vi "Periodic Tasks.vi"(8 "error in":errorcluster) -> ()   [LabVIEW 2012]
doc: "This VI runs in parallel to other tasks. It can contain as many user-defined periodic loops as you need. These can carry out PID or other sorts of timed response."
uses:
  <vilib>/Rock Robotics/SystemInterfaces/Utilities/FPGA_UtilitiesLED Source.ctl
  <vilib>/Rock Robotics/SystemInterfaces/Utilities/FPGA_UtilitiesLED State.ctl
  <vilib>/Rock Robotics/WPI/RobotDrive/WPI_RobotDriveGetSetRefNum.vi
  Robot Global Data.vi
  <vilib>/Rock Robotics/WPI/Joystick/WPI_JoystickGetSetRefNum.vi
  <vilib>/addons/control/pid/pid.llb/PID (DBL).vi
  <vilib>/addons/control/pid/NI_PID_pid.lvlib
panel:
  in  "setpoint 4":dbl=1500.0 format="%.2f"
  in  "setpoint 3":dbl=1500.0 format="%.2f"
  in  "PID gains 3":T1={"proportional gain (Kc)"=0.01, "integral time (Ti, min)"=0.0, "derivative time (Td, min)"=0.0}
  in  "PID gains 2":T1={"proportional gain (Kc)"=0.01, "integral time (Ti, min)"=0.0, "derivative time (Td, min)"=0.0}
  in  "PID gains":T1={"proportional gain (Kc)"=0.01, "integral time (Ti, min)"=0.0, "derivative time (Td, min)"=0.0}
  in  "setpoint":dbl=1500.0 format="%.2f"
  in  "setpoint 2":dbl=1500.0 format="%.2f"
  in  "Accel Rate":dbl=0.1
  in  "error in 2":errorcluster
  out "Sonar Distance Average":dbl
  out "Sonar Distance Output":dbl
  out "Sonar Voltage":dbl
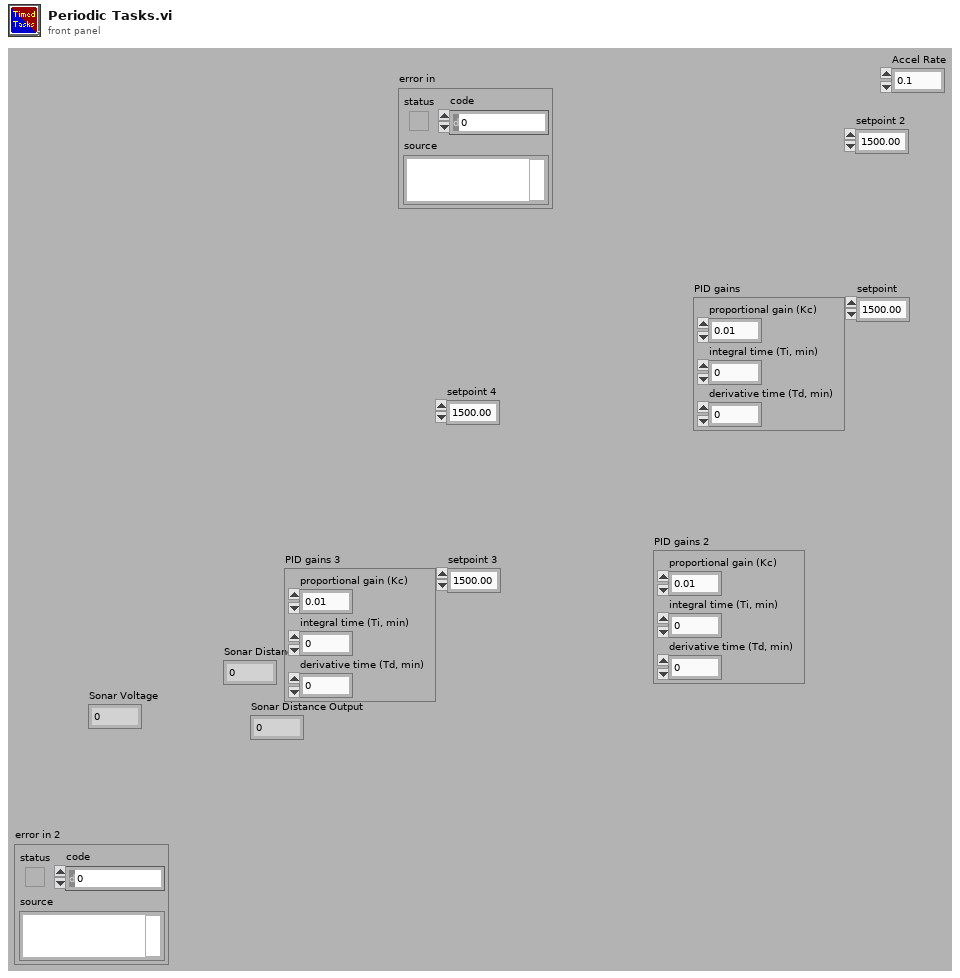
[diagram p1: front panel]
types:
  T1 = cluster{"proportional gain (Kc)":dbl, "integral time (Ti, min)":dbl, "derivative time (Td, min)":dbl}
  T2 = typedef "WPI_JoystickDevRef.ctl" = cluster{"Device":T3}
  T3 = typedef "WPI_JoystickDeviceEnum.ctl" = enum16{"USB 1", "USB 2", "USB 3", "USB 4", "Kinect 1", "Kinect 2"}
  T4 = typedef "WPI_RobotDriveDevRef.ctl" = cluster{"DevStatus":errorcluster, "Motors[]":T5[], "Square Inputs":bool, "Max Output":dbl, "Isochronous":bool}
  T5 = typedef "WPI_MotorControlDeviceRef.ctl" = cluster{"DeviceStatus":errorcluster, "Type":enum16{"PWM", "CAN"}, "PWM":cluster{"Digital Module":T6, "PWM Channel":T7, "DeadBand":T8}, "CAN":cluster{"Device Number":u8, "Control Mode":T9, "Semaphore":T10, "Max Vout":dbl}, "Invert":bool, "TransformRef":T11, "InvTransformRef":T11}
  T6 = typedef "FPGA_TypedefDigitalModule.ctl" = enum16{"Digital Module 1", "Digital Module 2"}
  T7 = typedef "FPGA_DIOPWMChannel.ctl" = enum8{"PWM 1", "PWM 2", "PWM 3", "PWM 4", "PWM 5", "PWM 6", "PWM 7", "PWM 8", "PWM 9", "PWM 10", "Invalid"}
  T8 = typedef "WPI_PWMDeadband.ctl" = cluster{"Name":string, "maxPositivePwm":i32, "minPositivePwm":i32, "centerPwm":i32, "maxNegativePwm":i32, "minNegativePwm":i32, "angularRange":u16}
  T9 = typedef "WPI_CANJaguar_ControlMode.ctl" = enum8{"Percent VBus", "Current", "Speed", "Position", "Voltage"}
  T10 = typedef "Semaphore RefNum" = refnum<k1>
  T11 = typedef "WPI_PWMTransform_ConPane.ctl" = refnum<vi>
  T12 = cluster{"JoystickDevRef":T2, "RobotDriveDevRef":T4, "RobotDriveDevRef":T4}
  T13 = cluster{"axis 1 (x)":dbl, "axis 2 (y)":dbl, "axis 3 (throttle)":dbl, "axis 4":dbl, "axis 5":dbl, "axis 6":dbl}
  T14 = typedef "WPI_AnalogChannelDevRef.ctl" = cluster{"DevStatus":errorcluster, "Analog Module":T15, "Analog Channel":T16}
  T15 = typedef "FPGA_TypedefAnalogModule.ctl" = enum16{"Analog Module 1", "Analog Module 2"}
  T16 = typedef "FPGA_AIChannel.ctl" = enum8{"AI 1", "AI 2", "AI 3", "AI 4", "AI 5", "AI 6", "AI 7", "AI 8", "Invalid"}
  T17 = typedef "WPI_DigitalOutputDevRef.ctl" = cluster{"Digital Module":T6, "DIO Channel":T18, "DevStatus":errorcluster}
  T18 = typedef "FPGA_DIOChannel.ctl" = enum8{"DIO 1", "DIO 2", "DIO 3", "DIO 4", "DIO 5", "DIO 6", "DIO 7", "DIO 8", "DIO 9", "DIO 10", "DIO 11", "DIO 12", "DIO 13", "DIO 14", "Invalid"}
  T19 = typedef "WPI_JoystickButtonState.ctl" = cluster{"Button 1":bool, "Button 2":bool, "Button 3":bool, "Button 4":bool, "Button 5":bool, "Button 6":bool, "Button 7":bool, "Button 8":bool, "Button 9":bool, "Button 10":bool, "Button 11":bool, "Button 12":bool}
  T20 = typedef "FPGA_UtilitiesLED State.ctl" = enum16{"Off", "On", "Toggle"}
  T21 = typedef "FPGA_UtilitiesLED Source.ctl" = enum16{"User LED", "FPGA LED"}
  T22 = typedef "WPI_EncoderDevRef.ctl" = cluster{"DevStatus":errorcluster, "EncoderIndex":T23, "CounterIndex":T24, "DistancePerCount":dbl, "Decoding Type":T25}
  T23 = typedef "FPGA_EncoderIdx.ctl" = enum8{"Enc 0", "Enc 1", "Enc 2", "Enc 3", "Invalid"}
  T24 = typedef "FPGA_CounterCtrSystemIndex.ctl" = enum8{"Ctr 0", "Ctr 1", "Ctr 2", "Ctr 3", "Ctr 4", "Ctr 5", "Ctr 6", "Ctr 7", "Invalid"}
  T25 = typedef "WPI_EncoderType.ctl" = enum16{"1x", "2x", "4x"}
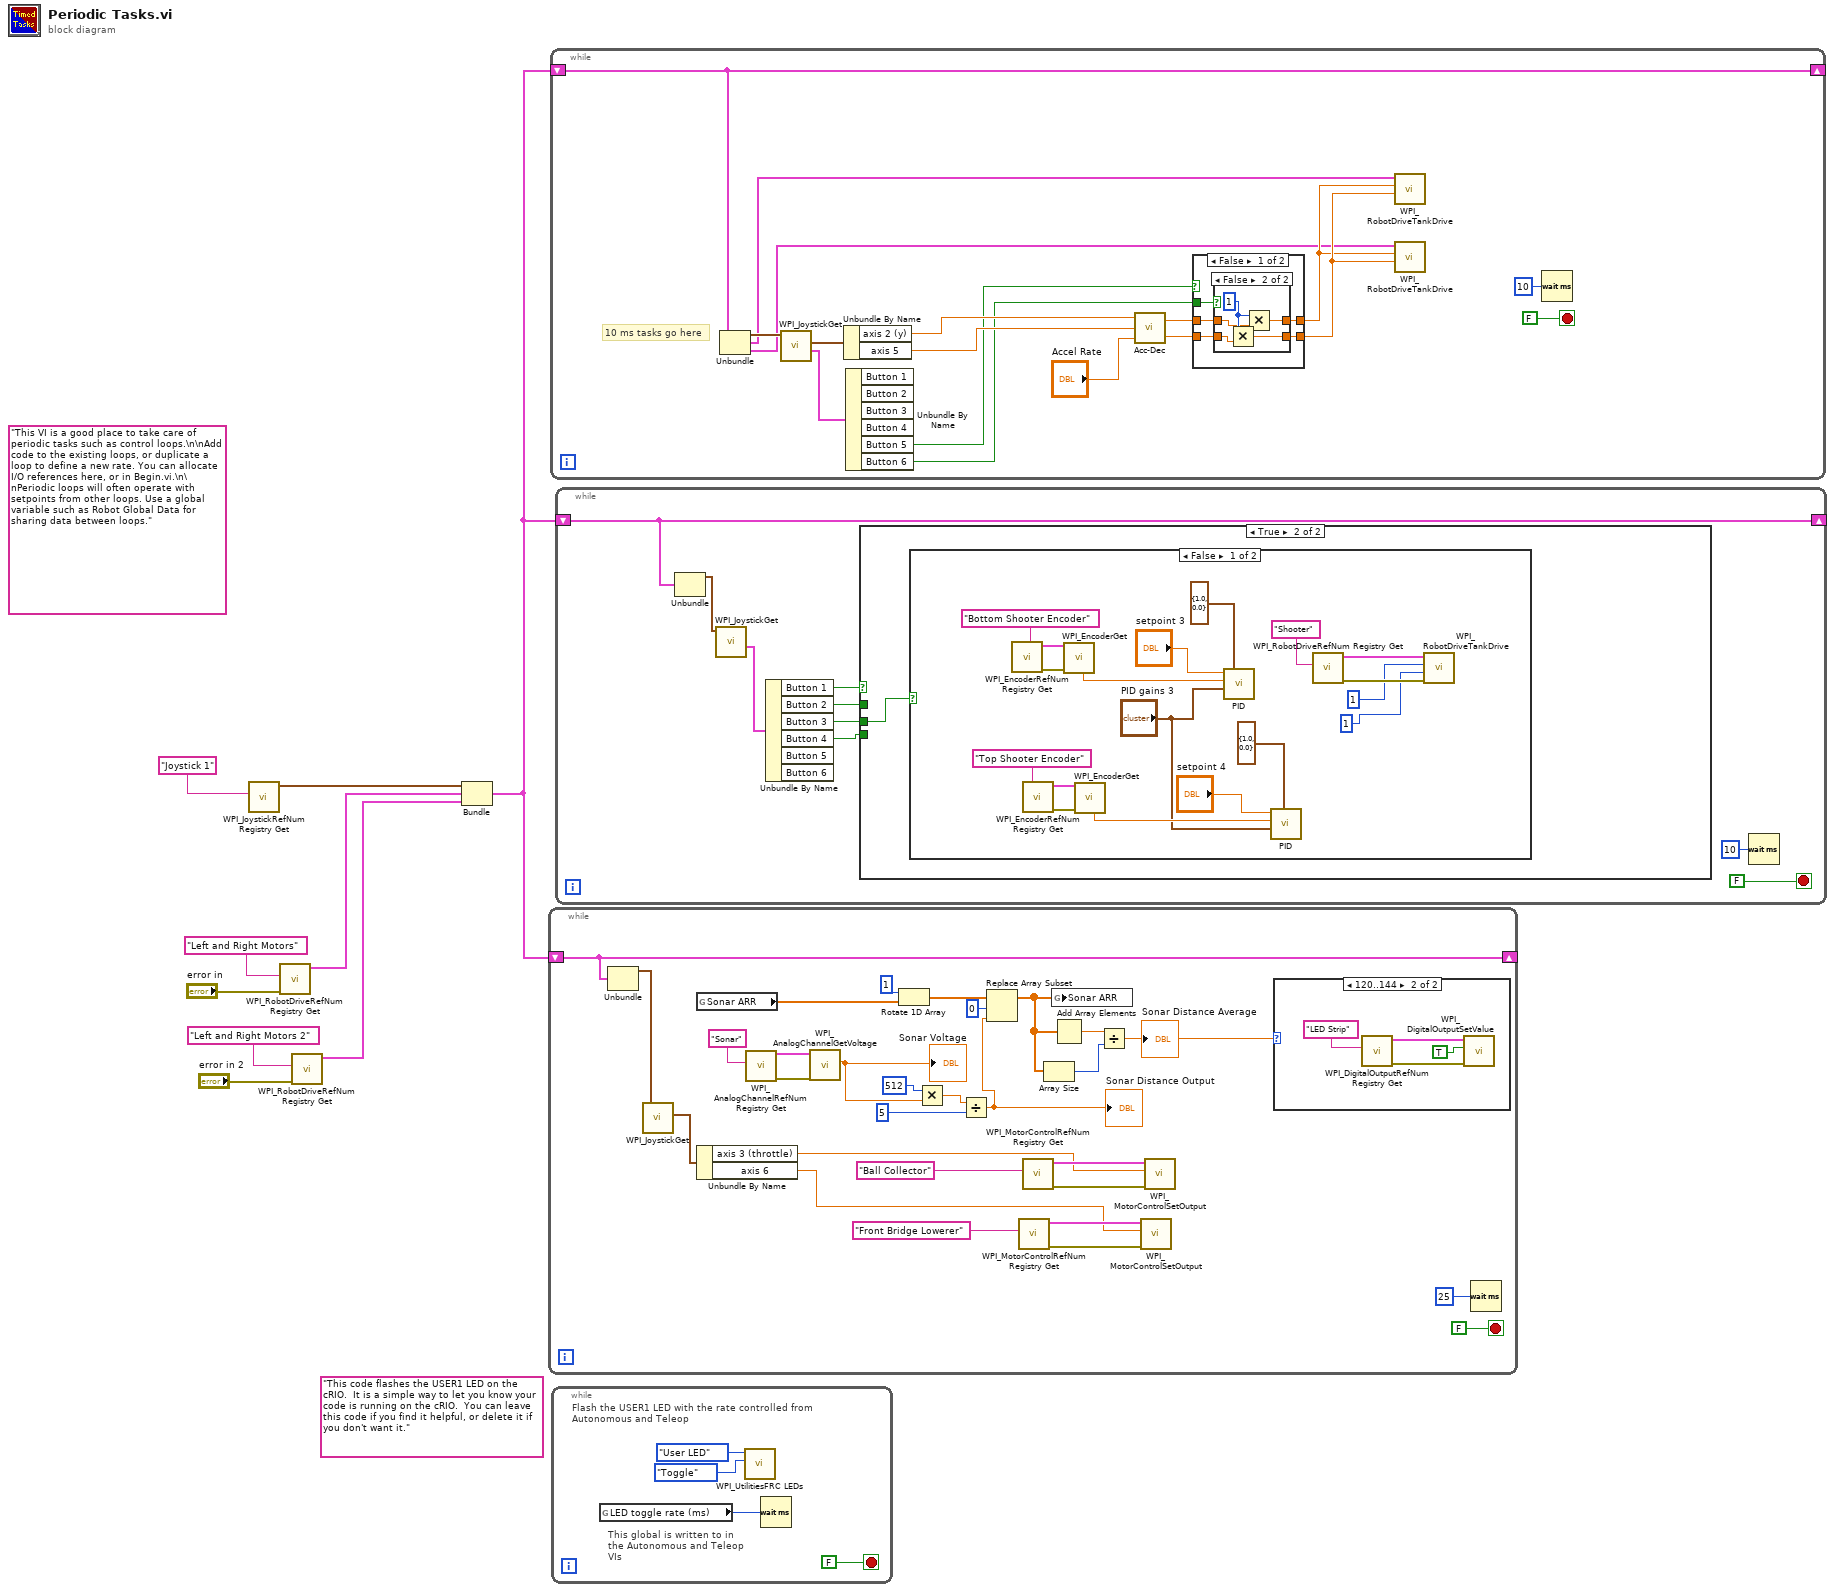
[diagram p0: block diagram]
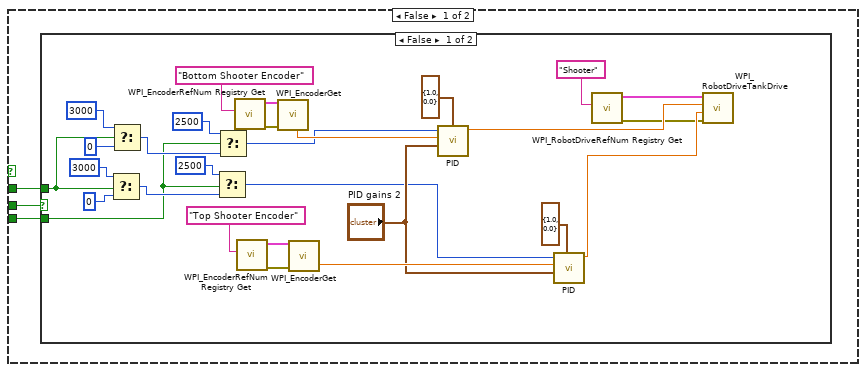
[diagram p2: hidden frame]
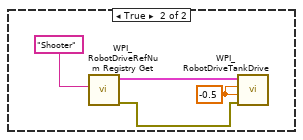
[diagram p3: hidden frame]
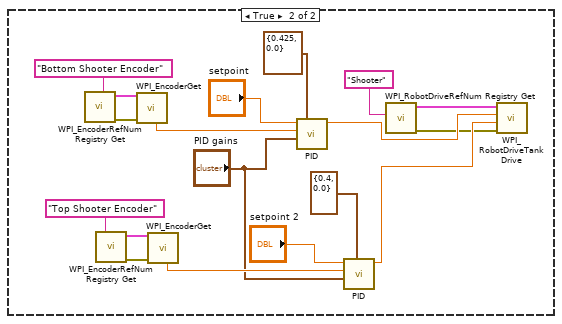
[diagram p4: hidden frame]
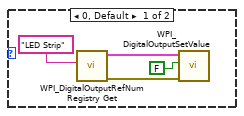
[diagram p5: hidden frame]
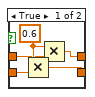
[diagram p6: hidden frame]
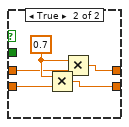
[diagram p7: hidden frame]
diagram:
  (unwired) "This code flashes the USER1 LED on the cRIO.  It is a simple way to let you know your code is running on the cRIO.  You can leave this code if you find it helpful, or delete it if you don't want it."
  (unwired) "This VI is a good place to take care of periodic tasks such as control loops.\n\nAdd code to the existing loops, or duplicate a loop to define a new rate. You can allocate I/O references here, or in Begin.vi.\n\nPeriodic loops will often operate with setpoints from other loops. Use a global variable such as Robot Global Data for sharing data between loops."
  n1 = call <vilib>:"WPI_JoystickRefNum Registry Get.vi"("refnum name"="Joystick 1") -> ("JoystickDevRef"=w7:T2)  [unwired: 1 in, 9 out]
  n2 = call <vilib>:"WPI_RobotDriveRefNum Registry Get.vi"("error in (no error)"="error in", "refnum name"="Left and Right Motors") -> ("RobotDriveDevRef"=w6:T4)  [unwired: 9 out]
  n3 = call <vilib>:"WPI_RobotDriveRefNum Registry Get.vi"("error in (no error)"="error in 2", "refnum name"="Left and Right Motors 2") -> ("RobotDriveDevRef"=w2:T4)  [unwired: 9 out]
  n4 = Bundle("JoystickDevRef"=w7, "RobotDriveDevRef"=w6, "RobotDriveDevRef"=w2) -> (w1:T12)  [unwired: 1 out]
  n5 = while {
    shift-right: [w20] -> _
    shift-left: w1 -> [w20]
    stop <- FALSE stop-if-true
    n6 = Unbundle(w20) -> ("JoystickDevRef"=w18:T2)  [unwired: 2 out]
    n7 = call <vilib>:"WPI_JoystickGet.vi"("JoystickDevRef"=w18) -> ("Axes"=w19:T13)  [unwired: 1 in, 5 out]
    n8 = global read "Robot Global Data.vi" "Sonar ARR"() -> (w31:dbl[])
    n9 = Unbundle By Name(w19) -> ("axis 3 (throttle)"=w10:dbl, "axis 6"=w14:dbl)
    n10 = call <vilib>:"WPI_AnalogChannelRefNum Registry Get.vi"("refnum name"="Sonar") -> ("error out"=w23:errorcluster, "AIDeviceRef"=w33:T14)  [unwired: 9 in]
    n11 = call <vilib>:"WPI_AnalogChannelGetVoltage.vi"("error in (no error)"=w23, "AIDeviceRef"=w33) -> ("Voltage"=w32:dbl)  [unwired: 7 in, 2 out]
    "Sonar Voltage" <- w32
    n12 = Rotate 1D Array(1:w31, 2:1) -> (0:w29:dbl[])
    n13 = Multiply(x=512, y=w32) -> (x*y=w35:dbl)
    n14 = Divide(x=w35, y=5) -> (x/y=w28:dbl)
    "Sonar Distance Output" <- w28
    n15 = Replace Array Subset(array=w29, new element=w28, index=0) -> (w25:dbl[])
    n16 = call <vilib>:"WPI_MotorControlRefNum Registry Get.vi"("refnum name"="Front Bridge Lowerer") -> ("error out"=w16:errorcluster, "MotorControlDevRef"=w15:T5)  [unwired: 9 in]
    n17 = call <vilib>:"WPI_MotorControlRefNum Registry Get.vi"("refnum name"="Ball Collector") -> ("error out"=w12:errorcluster, "MotorControlDevRef"=w11:T5)  [unwired: 9 in]
    n18 = Array Size(array=w25) -> (size(s)=w24:i32)
    n19 = global write "Robot Global Data.vi" "Sonar ARR"(w25) -> ()
    n20 = Add Array Elements(numeric array=w25) -> (sum=w26:dbl)
    n21 = Divide(x=w26, y=w24) -> (x/y=w22:dbl)
    "Sonar Distance Average" <- w22
    n22 = call <vilib>:"WPI_MotorControlSetOutput.vi"("error in (no error)"=w16, "Output"=w14, "MotorControlDevRef"=w15) -> ()  [unwired: 6 in, 3 out]
    n23 = call <vilib>:"WPI_MotorControlSetOutput.vi"("error in (no error)"=w12, "Output"=w10, "MotorControlDevRef"=w11) -> ()  [unwired: 6 in, 3 out]
    n24 = case shown="120..144" w22 {
      frame 0, Default {
        n25 = call <vilib>:"WPI_DigitalOutputRefNum Registry Get.vi"("refnum name"="LED Strip") -> ("error out"=w40:errorcluster, "DigitalOutputDevRef"=w41:T17)  [unwired: 9 in]
        n26 = call <vilib>:"WPI_DigitalOutputSetValue.vi"("error in (no error)"=w40, "Value"=FALSE, "DigitalOutputDevRef"=w41) -> ()  [unwired: 7 in, 2 out]
      }
      frame 120..144 {
        n27 = call <vilib>:"WPI_DigitalOutputRefNum Registry Get.vi"("refnum name"="LED Strip") -> ("error out"=w44:errorcluster, "DigitalOutputDevRef"=w45:T17)  [unwired: 9 in]
        n28 = call <vilib>:"WPI_DigitalOutputSetValue.vi"("error in (no error)"=w44, "Value"=TRUE, "DigitalOutputDevRef"=w45) -> ()  [unwired: 7 in, 2 out]
      }
    }
    n29 = Wait (ms)(milliseconds to wait=u32 25) -> ()  [unwired: 1 out]
  }
  n30 = while {
    shift-right: [w61] -> _
    shift-left: w1 -> [w61]
    stop <- FALSE stop-if-true
    # "10 ms tasks go here"
    n31 = Unbundle(w61) -> ("JoystickDevRef"=w58:T2, "RobotDriveDevRef"=w55:T4, "RobotDriveDevRef"=w54:T4)
    n32 = call <vilib>:"WPI_JoystickGet.vi"("JoystickDevRef"=w58) -> ("Buttons"=w59:T19, "Axes"=w60:T13)  [unwired: 1 in, 4 out]
    n33 = Unbundle By Name(w60) -> ("axis 2 (y)"=w51:dbl, "axis 5"=w52:dbl)
    n34 = Unbundle By Name(w59) -> ("Button 5"=w47:bool, "Button 6"=w48:bool)  [unwired: 4 out]
    n35 = call "Acc-Dec.vi"("Acc Rate"="Accel Rate", "Y-Input 2"=w52, "Y-Input 1"=w51) -> ("Y-Output 2"=w49:dbl, "Y-Output 1"=w50:dbl)
    n36 = case shown="False" w47 {
      tunnel: [w68 w79] -> w57
      tunnel: [w67 w80] -> w56
      tunnel: w50 -> [w66 w81]
      tunnel: w49 -> [w65 w82]
      tunnel: w48 -> [w64 _]
      frame False {
        n37 = case shown="False" w64 {
          tunnel: [w71 w76] -> w67
          tunnel: w66 -> [w69 w74]
          tunnel: [w73 w78] -> w68
          tunnel: w65 -> [w72 w77]
          frame True {
            w70 = 0.6
            n38 = Multiply(x=w70, y=w72) -> (x*y=w73:dbl)
            n39 = Multiply(x=w70, y=w69) -> (x*y=w71:dbl)
          }
          frame False {
            w75 = 1
            n40 = Multiply(x=w75, y=w77) -> (x*y=w78:dbl)
            n41 = Multiply(x=w75, y=w74) -> (x*y=w76:dbl)
          }
        }
      }
      frame True {
        w83 = 0.7
        n42 = Multiply(x=w83, y=w82) -> (x*y=w79:dbl)
        n43 = Multiply(x=w83, y=w81) -> (x*y=w80:dbl)
      }
    }
    n44 = call <vilib>:"WPI_RobotDriveTankDrive.vi"("Right axis value"=w57, "Left axis value"=w56, "RobotDriveDevRef"=w55) -> ()  [unwired: 6 in, 3 out]
    n45 = call <vilib>:"WPI_RobotDriveTankDrive.vi"("Right axis value"=w57, "Left axis value"=w56, "RobotDriveDevRef"=w54) -> ()  [unwired: 6 in, 3 out]
    n46 = Wait (ms)(milliseconds to wait=u32 10) -> ()  [unwired: 1 out]
  }
  n47 = while {
    stop <- FALSE stop-if-true
    # "This global is written to in the Autonomous and Teleop VIs"
    # "Flash the USER1 LED with the rate controlled from Autonomous and Teleop"
    n48 = global read "Robot Global Data.vi" "LED toggle rate (ms)"() -> (w84:u32)
    n49 = call <vilib>:"WPI_UtilitiesFRC LEDs.vi"("State"=FPGA_UtilitiesLED_State."Toggle", "LED Type"=FPGA_UtilitiesLED_Source."User LED") -> ()  [unwired: 1 in, 9 out]
    n50 = Wait (ms)(milliseconds to wait=w84) -> ()  [unwired: 1 out]
  }
  n51 = while {
    shift-right: [w96] -> _
    shift-left: w1 -> [w96]
    stop <- FALSE stop-if-true
    n52 = Unbundle(w96) -> ("JoystickDevRef"=w94:T2)  [unwired: 2 out]
    n53 = call <vilib>:"WPI_JoystickGet.vi"("JoystickDevRef"=w94) -> ("Buttons"=w95:T19)  [unwired: 1 in, 5 out]
    n54 = Unbundle By Name(w95) -> ("Button 1"=w93:bool, "Button 2"=w89:bool, "Button 3"=w92:bool, "Button 4"=w88:bool)  [unwired: 2 out]
    n55 = case shown="True" w93 {
      tunnel: w92 -> [w99 w132]
      tunnel: w89 -> [w98 _]
      tunnel: w88 -> [w97 _]
      frame False {
        n56 = case shown="False" w99 {
          tunnel: w98 -> [w108 _]
          tunnel: w97 -> [w103 _]
          frame False {
            n57 = Select(t=3000, s=w108, f=0) -> (s? t:f=w104:i32)
            n58 = Select(t=3000, s=w108, f=0) -> (s? t:f=w105:i32)
            n59 = Select(t=2500, s=w103, f=w104) -> (s? t:f=w102:i32)
            n60 = Select(t=2500, s=w103, f=w105) -> (s? t:f=w101:i32)
            n61 = call <vilib>:"WPI_EncoderRefNum Registry Get.vi"("refnum name"="Bottom Shooter Encoder") -> ("error out"=w120:errorcluster, "EncoderDevRef"=w121:T22)  [unwired: 9 in]
            n62 = call <vilib>:"WPI_EncoderRefNum Registry Get.vi"("refnum name"="Top Shooter Encoder") -> ("error out"=w123:errorcluster, "EncoderDevRef"=w124:T22)  [unwired: 9 in]
            n63 = call <vilib>:"WPI_EncoderGet.vi"("error in (no error)"=w120, "EncoderDevRef"=w121) -> ("Rate"=w118:dbl)  [unwired: 4 in, 5 out]
            n64 = call <vilib>:"WPI_EncoderGet.vi"("error in (no error)"=w123, "EncoderDevRef"=w124) -> ("Rate"=w117:dbl)  [unwired: 4 in, 5 out]
            n65 = call-poly <vilib>:"PID.vi"("output range"=cluster{"output high":dbl, "output low":dbl} {"output high"=1.0, "output low"=0.0}, "PID gains"="PID gains 2", "process variable"=w118, "setpoint"=w101) -> ("output"=w115:dbl)  [unwired: 6 in, 1 out]
            n66 = call-poly <vilib>:"PID.vi"("output range"=cluster{"output high":dbl, "output low":dbl} {"output high"=1.0, "output low"=0.0}, "PID gains"="PID gains 2", "process variable"=w117, "setpoint"=w102) -> ("output"=w116:dbl)  [unwired: 6 in, 1 out]
            n67 = call <vilib>:"WPI_RobotDriveRefNum Registry Get.vi"("refnum name"="Shooter") -> ("error out"=w100:errorcluster, "RobotDriveDevRef"=w127:T4)  [unwired: 1 in, 8 out]
            n68 = call <vilib>:"WPI_RobotDriveTankDrive.vi"("error in (no error)"=w100, "Right axis value"=w116, "Left axis value"=w115, "RobotDriveDevRef"=w127) -> ()  [unwired: 5 in, 3 out]
          }
          frame True {
            w129 = -0.5
            n69 = call <vilib>:"WPI_RobotDriveRefNum Registry Get.vi"("refnum name"="Shooter") -> ("error out"=w128:errorcluster, "RobotDriveDevRef"=w130:T4)  [unwired: 1 in, 8 out]
            n70 = call <vilib>:"WPI_RobotDriveTankDrive.vi"("error in (no error)"=w128, "Right axis value"=w129, "Left axis value"=w129, "RobotDriveDevRef"=w130) -> ()  [unwired: 5 in, 3 out]
          }
        }
      }
      frame True {
        n71 = case shown="False" w132 {
          frame False {
            n72 = call <vilib>:"WPI_EncoderRefNum Registry Get.vi"("refnum name"="Bottom Shooter Encoder") -> ("error out"=w140:errorcluster, "EncoderDevRef"=w141:T22)  [unwired: 9 in]
            n73 = call <vilib>:"WPI_EncoderRefNum Registry Get.vi"("refnum name"="Top Shooter Encoder") -> ("error out"=w143:errorcluster, "EncoderDevRef"=w144:T22)  [unwired: 9 in]
            n74 = call <vilib>:"WPI_EncoderGet.vi"("error in (no error)"=w140, "EncoderDevRef"=w141) -> ("Rate"=w138:dbl)  [unwired: 4 in, 5 out]
            n75 = call <vilib>:"WPI_EncoderGet.vi"("error in (no error)"=w143, "EncoderDevRef"=w144) -> ("Rate"=w137:dbl)  [unwired: 4 in, 5 out]
            n76 = call-poly <vilib>:"PID.vi"("output range"=cluster{"output high":dbl, "output low":dbl} {"output high"=1.0, "output low"=0.0}, "PID gains"="PID gains 3", "process variable"=w138, "setpoint"="setpoint 3") -> ()  [unwired: 6 in, 2 out]
            n77 = call-poly <vilib>:"PID.vi"("output range"=cluster{"output high":dbl, "output low":dbl} {"output high"=1.0, "output low"=0.0}, "PID gains"="PID gains 3", "process variable"=w137, "setpoint"="setpoint 4") -> ()  [unwired: 6 in, 2 out]
            n78 = call <vilib>:"WPI_RobotDriveRefNum Registry Get.vi"("refnum name"="Shooter") -> ("error out"=w135:errorcluster, "RobotDriveDevRef"=w150:T4)  [unwired: 1 in, 8 out]
            n79 = call <vilib>:"WPI_RobotDriveTankDrive.vi"("error in (no error)"=w135, "Right axis value"=1, "Left axis value"=1, "RobotDriveDevRef"=w150) -> ()  [unwired: 5 in, 3 out]
          }
          frame True {
            n80 = call <vilib>:"WPI_EncoderRefNum Registry Get.vi"("refnum name"="Bottom Shooter Encoder") -> ("error out"=w158:errorcluster, "EncoderDevRef"=w159:T22)  [unwired: 9 in]
            n81 = call <vilib>:"WPI_EncoderRefNum Registry Get.vi"("refnum name"="Top Shooter Encoder") -> ("error out"=w161:errorcluster, "EncoderDevRef"=w162:T22)  [unwired: 9 in]
            n82 = call <vilib>:"WPI_EncoderGet.vi"("error in (no error)"=w158, "EncoderDevRef"=w159) -> ("Rate"=w156:dbl)  [unwired: 4 in, 5 out]
            n83 = call <vilib>:"WPI_EncoderGet.vi"("error in (no error)"=w161, "EncoderDevRef"=w162) -> ("Rate"=w155:dbl)  [unwired: 4 in, 5 out]
            n84 = call-poly <vilib>:"PID.vi"("output range"=cluster{"output high":dbl, "output low":dbl} {"output high"=0.425, "output low"=0.0}, "PID gains"="PID gains", "process variable"=w156, "setpoint"="setpoint") -> ("output"=w153:dbl)  [unwired: 6 in, 1 out]
            n85 = call-poly <vilib>:"PID.vi"("output range"=cluster{"output high":dbl, "output low":dbl} {"output high"=0.4, "output low"=0.0}, "PID gains"="PID gains", "process variable"=w155, "setpoint"="setpoint 2") -> ("output"=w154:dbl)  [unwired: 6 in, 1 out]
            n86 = call <vilib>:"WPI_RobotDriveRefNum Registry Get.vi"("refnum name"="Shooter") -> ("error out"=w151:errorcluster, "RobotDriveDevRef"=w168:T4)  [unwired: 1 in, 8 out]
            n87 = call <vilib>:"WPI_RobotDriveTankDrive.vi"("error in (no error)"=w151, "Right axis value"=w154, "Left axis value"=w153, "RobotDriveDevRef"=w168) -> ()  [unwired: 5 in, 3 out]
          }
        }
      }
    }
    n88 = Wait (ms)(milliseconds to wait=u32 10) -> ()  [unwired: 1 out]
  }
